vi "DSF.Engine.Framework.Rx.Inline.Wait.vi"(8 "error in (no error)":errorcluster, 11 "Framework in":refnum<class "DSF.Engine.Framework.lvclass">) -> (0 "error out":errorcluster, 3 "Framework out":refnum<class "DSF.Engine.Framework.lvclass">)   [LabVIEW 2017, in "DSF.Engine.lvlib" / "DSF.Engine.Framework.lvclass"]
uses:
  DSF.Engine.Framework.lvclass
  DSF.Engine.Framework.lvclass/DSF.Engine.Framework.ctl
  Plugin/DSF.Engine.Plugin.lvclass/DSF.Engine.Plugin.ctl
  Timing/DSF.Engine.Timing.lvclass/DSF.Engine.Timing.ctl
  Transfer/DSF.Engine.Transfer Group.lvclass/DSF.Engine.Transfer Group.ctl
  Debug/DSF.Engine.Debug Flags.lvclass/DSF.Engine.Debug Flags.ctl
  Debug/DSF.Engine.Debug Flags.FIFO.lvclass/DSF.Engine.Debug Flags.FIFO.ctl
  Transfer/DSF.Engine.Transfer.lvclass/DSF.Engine.Transfer.ctl
  Transfer/DSF.Engine.Transfer Group.Get Timing.vi
  Timing/DSF.Engine.Timing.Get Iteration.vi
  Transfer/DSF.Engine.Transfer Group.Retrieve from FIFO.vi
  Transfer/DSF.Engine.Transfer Group.Move Channels to Engine.vi
  Plugin/DSF.Engine.Plugin.Get Timing.vi
  Timing/DSF.Engine.Timing.Is Active Cycle.vi
  Transfer/DSF.Engine.Transfer Group.Return FIFO.Read.vi
  Transfer/DSF.Engine.Transfer Group.Get Transfers.vi
  Transfer/DSF.Engine.Transfer.Get Inline Buffer.vi
  Transfer/DSF.Engine.Transfer.Get Intermediate Buffer.vi
  Timing/DSF.Engine.Timing.Get Decimation.vi
  Timing/DSF.Engine.Timing.Get Offset.vi
  Transfer/DSF.Engine.Transfer Group.Get Return FIFO.vi
  Transfer/DSF.Engine.Transfer Group.Get Debug Flags.vi
  Debug/DSF.Engine.Debug Flags.Get FIFO Flags.vi
  Debug/DSF.Engine.Debug Flags.FIFO.Get Infinite Timeouts.vi
  Built/Memory/Memory Manager.lvlibp/1abvi3w/vi.lib/National Instruments/Memory Manager/Classes/Pointer/Memory.Pointer.Copy All.vi
  Transfer/DSF.Engine.Transfer Group.Errors.vi
  Transfer/DSF.Engine.Transfer Group.Errors.Return Timeout.vi
  Plugin/DSF.Engine.Plugin.lvclass
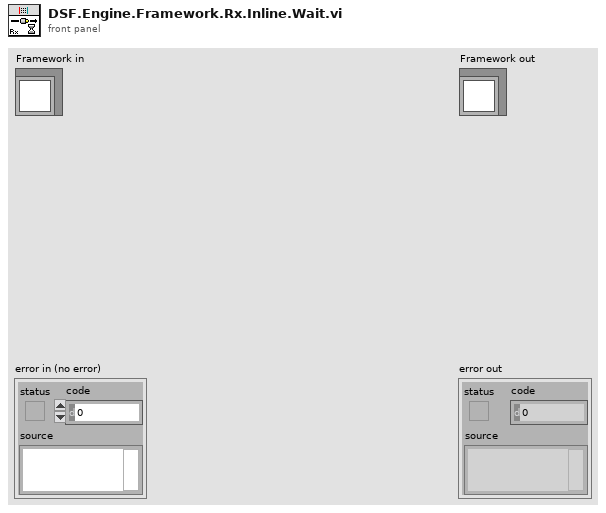
[diagram p1: front panel]
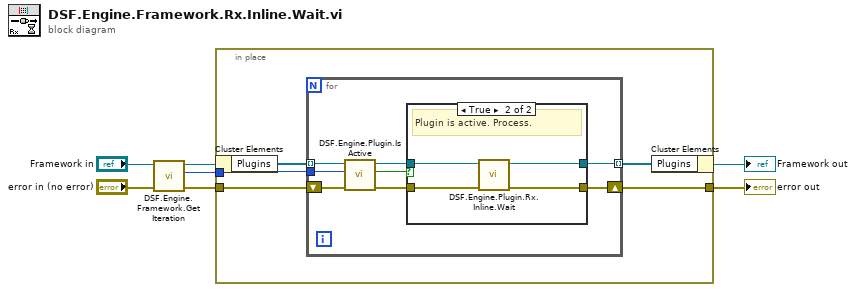
[diagram p0: block diagram]
diagram:
  n1 = call "DSF.Engine.Framework.Get Iteration.vi"("Framework in"="Framework in") -> ("iteration"=w4:u64, "Framework out"=w1:refnum<class "DSF.Engine.Framework.lvclass">)  [unwired: 9 in]
  n2 = in-place {
    in-place-border: "error in (no error)" -> [w11]
    in-place-border: [w10] -> w5
    in-place-border: w4 -> [w9]
    n3 = in-place-cluster #1(w1) -> ("Plugins"=w8:refnum<class "DSF.Engine.Plugin.lvclass">[])
    n4 = for {
      tunnel: w8 -> [w15] mode=indexing
      tunnel: [w18] -> w7 mode=indexing
      shift-right: [w17] -> w10
      shift-left: w11 -> [w16]
      tunnel: w9 -> [w12]
      n5 = call "DSF.Engine.Plugin.Is Active.vi"("cycle count"=w12, "Plugin in"=w15) -> ("active this cycle?"=w13:bool, "Plugin out"=w14:refnum<class "DSF.Engine.Plugin.lvclass">)  [unwired: 8 in]
      n6 = case shown="True" w13 {
        tunnel: w14 -> [w20 w24]
        tunnel: [w20 w21] -> w18
        tunnel: [w19 w22] -> w17
        tunnel: w16 -> [w19 w23]
        frame False {
          # "Plugin is not active. Skip."
        }
        frame True {
          # "Plugin is active. Process."
          n7 = call "DSF.Engine.Plugin.Rx.Inline.Wait.vi"("error in (no error)"=w23, "Plugin in"=w24) -> ("error out"=w22:errorcluster, "Plugin out"=w21:refnum<class "DSF.Engine.Plugin.lvclass">)  [unwired: 8 in]
        }
      }
    }
    n8 = in-place-cluster #1("Plugins"=w7) -> (→"Framework out":refnum<class "DSF.Engine.Framework.lvclass">)
  }
  "error out" <- w5
